vi "ODX_Query XML for Flashdata.vi"(8 "error in (no error)":errorcluster, 10 "XML document":string="<?xml version=\"1.0\" encoding=\"ISO-8859-1\"?>\n<bookstore>\n<book ISBN=\"978-0545128285\">\n  <title lang=\"en\">The Tales of Beedle the Bard</title>\n  <author>J. K. Rowling</author>\n  <year>2008</year>\n  <price>12.99</price>\n</book>\n<book ISBN=\"978-0316160209\">\n  <title lang=\"en\">Eclipse</title>\n  <author>Stephenie Meyer</author>\n  <year>2007</year>\n  <price>19.99</price>\n</book>\n<book ISBN=\"978-0316067928\">\n  <title lang=\"en\">Breaking Dawn</title>\n  <author>Stephenie Meyer</author>\n  <year>2008</year>\n  <price>22.99</price>\n</book>\n<book ISBN=\"978-0316017923\">\n  <title lang=\"en\">Outliers: The Story of Success</title>\n  <author>Malcolm Gladwell</author>\n  <year>2008</year>\n  <price>27.99</price>\n</book>\n<book ISBN=\"978-0596007645\">\n  <title lang=\"en\">XML in a Nutshell</title>\n  <author>Elliotte Rusty Harold</author>\n  <author>W. Scott Means</author>\n  <year>2004</year>\n  <price>39.95</price>\n</book>\n</bookstore>", 11 "XPath expression":string="/bookstore/book/title") -> (0 "error out":errorcluster, 1 "Result Array":string[](array[string]))   [LabVIEW 2012]
doc: "This example demonstrates how to query an XML document by using an XPath expression and returns all the nodes that match the XPath expression."
uses:
  <resource>/objmgr/DOMUserDefRef.rc
  <vilib>/xml/NI_XML.lvlib
  <vilib>/xml/Close Reference(Node).vi
panel:
  # "This example demonstrates how to query an XML document by using an XPath expression and returns all the nodes that \nmatch the XPath expression."
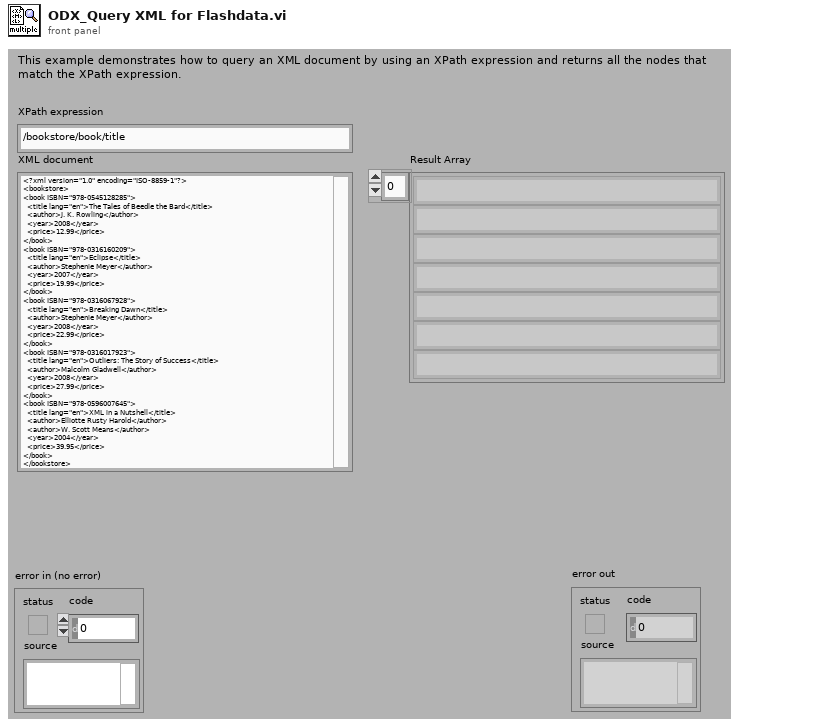
[diagram p1: front panel]
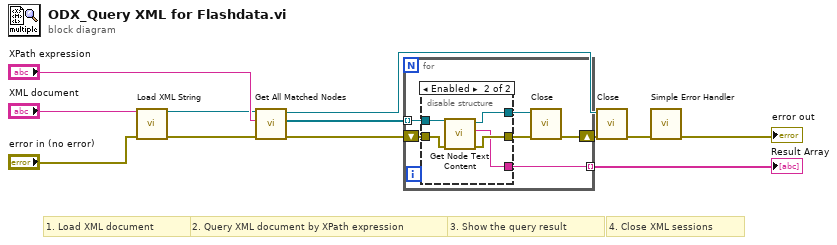
[diagram p0: block diagram]
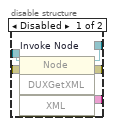
[diagram p2: hidden frame]
diagram:
  # "4. Close XML sessions"
  # "3. Show the query result"
  # "2. Query XML document by XPath expression"
  # "1. Load XML document"
  n1 = call <vilib>:"Load XML String.vi"("XML string"="XML document", "error in (no error)"="error in (no error)") -> ("DOM document out"=w7:refnum<k20>, "error out"=w9:errorcluster)  [unwired: 12 out]
  n2 = call <vilib>:"Get All Matched Nodes.vi"("error in (no error)"=w9, "XPath expression"="XPath expression", "node in"=w7) -> ("error out"=w10:errorcluster, "node result array"=w11:refnum<k20>[], "node out"=w5:refnum<k20>)  [unwired: 6 out]
  n3 = for {
    tunnel: w11 -> [w14] mode=indexing
    shift-right: [w16] -> w6
    shift-left: w10 -> [w15]
    tunnel: [w13] -> w3 mode=indexing
    n4 = disable-structure shown="Enabled" {
      disable-tunnel: [w23 w25] -> w18
      disable-tunnel: [w22 w27] -> w17
      disable-tunnel: w15 -> [w21 w26]
      disable-tunnel: w14 -> [w20 w28]
      disable-tunnel: [w19 w24] -> w13
      frame Disabled {
        n5 = invoke on="Invoke Node" class="Node" method="DUXGetXML"(reference=w20, error in=w21) -> (reference out=w22:refnum<k20>, error out=w23:errorcluster, "XML"=w19:string)  [unwired: 2 in, 1 out]
      }
      frame Enabled {
        n6 = call <vilib>:"Get Node Text Content.vi"("error in (no error)"=w26, "node in"=w28) -> ("error out"=w25:errorcluster, "node text"=w24:string, "node out"=w27:refnum<k20>)  [unwired: 7 in]
      }
    }
    n7 = call-poly <vilib>:"Close.vi"("error in (no error)"=w18, "node"=w17) -> ("error out"=w16:errorcluster)  [unwired: 7 out]
  }
  "Result Array" <- w3
  n8 = call-poly <vilib>:"Close.vi"("error in (no error)"=w6, "node"=w5) -> ("error out"=w4:errorcluster)  [unwired: 7 out]
  n9 = call <vilib>:"Simple Error Handler.vi"("error in (no error)"=w4) -> ("error out"=→"error out":errorcluster)  [unwired: 1 in, 7 out]
